vi "_readAppArgs.vi"(8 "error in (no error)":errorcluster, 11 "LVAutomationListener in":refnum<class "LVAutomationListener.lvclass">) -> (0 "error out":errorcluster, 3 "LVAutomationListener out":refnum<class "LVAutomationListener.lvclass">)   [LabVIEW 2013, in "LVAutomationListener.lvlib" / "LVAutomationListener.lvclass"]
doc: "Read the configuration file (if it exists) for values that will control this run of the application."
uses:
  LVAutomationListener.lvclass
  LVAutomationListener.lvclass/LVAutomationListener.ctl
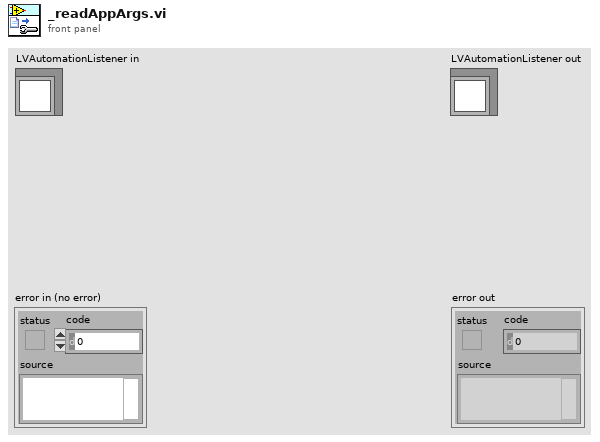
[diagram p1: front panel]
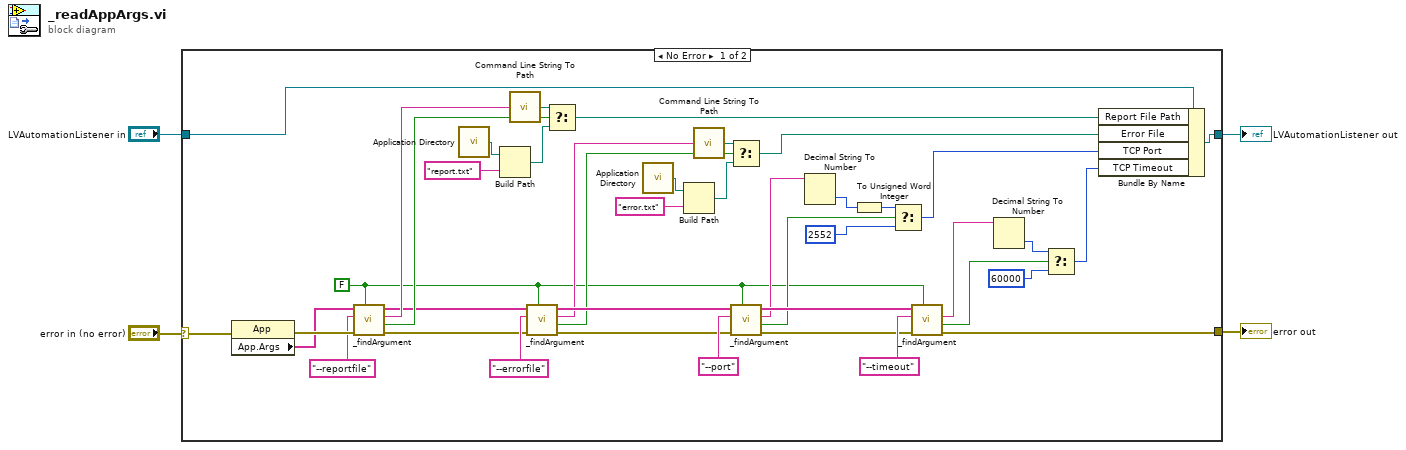
[diagram p0: block diagram]
diagram:
  n1 = case shown="No Error" "error in (no error)" {
    selector: "error in (no error)" -> [w46 w48]
    tunnel: [w21 w48] -> w3
    tunnel: [w43 w47] -> w1
    tunnel: "LVAutomationListener in" -> [w38 w47]
    frame No Error {
      w5 = FALSE ("Error If Not Found")
      n2 = property class="App"(error in=w46) -> (error out=w45:errorcluster, "App.Args"=w39:string[])  [unwired: 1 in, 1 out]
      n3 = call "_findArgument.vi"("Error If Not Found"=w5, "error in (no error)"=w45, "Argument"="--reportfile", "Arguments In"=w39) -> ("error out"=w15:errorcluster, "Found"=w40:bool, "Value"=w37:string, "Arguments Out"=w16:string[])  [unwired: 4 in]
      n4 = call <vilib>:"Application Directory.vi"() -> ("Application Directory"=w35:path)
      n5 = Build Path(base path=w35, name or relative path="report.txt") -> (appended path=w34:path)
      n6 = call <vilib>:"Command Line String To Path.vi"("string"=w37) -> ("path"=w36:path)
      n7 = call "_findArgument.vi"("Error If Not Found"=w5, "error in (no error)"=w15, "Argument"="--errorfile", "Arguments In"=w16) -> ("error out"=w13:errorcluster, "Found"=w7:bool, "Value"=w8:string, "Arguments Out"=w14:string[])  [unwired: 4 in]
      n8 = Select(t=w36, s=w40, f=w34) -> (s? t:f=w33:path)
      n9 = call <vilib>:"Application Directory.vi"() -> ("Application Directory"=w10:path)
      n10 = Build Path(base path=w10, name or relative path="error.txt") -> (appended path=w9:path)
      n11 = call <vilib>:"Command Line String To Path.vi"("string"=w8) -> ("path"=w11:path)
      n12 = Select(t=w11, s=w7, f=w9) -> (s? t:f=w6:path)
      n13 = call "_findArgument.vi"("Error If Not Found"=w5, "error in (no error)"=w13, "Argument"="--port", "Arguments In"=w14) -> ("error out"=w30:errorcluster, "Found"=w29:bool, "Value"=w28:string, "Arguments Out"=w31:string[])  [unwired: 4 in]
      n14 = Decimal String To Number(string=w28) -> (number=w18:i32)  [unwired: 2 in, 1 out]
      n15 = To Unsigned Word Integer(number=w18) -> (unsigned 16bit integer=w19:u16)
      n16 = Select(t=w19, s=w29, f=u16 2552) -> (s? t:f=w26:u16)
      n17 = call "_findArgument.vi"("Error If Not Found"=w5, "error in (no error)"=w30, "Argument"="--timeout", "Arguments In"=w31) -> ("error out"=w21:errorcluster, "Found"=w22:bool, "Value"=w23:string)  [unwired: 4 in, 1 out]
      n18 = Decimal String To Number(string=w23) -> (number=w25:i32)  [unwired: 2 in, 1 out]
      n19 = Select(t=w25, s=w22, f=60000) -> (s? t:f=w20:i32)
      n20 = Bundle By Name(cluster=w38, "Report File Path"=w33, "Error File"=w6, "TCP Port"=w26, "TCP Timeout"=w20) -> (w43:refnum<class "LVAutomationListener.lvclass">)
    }
    frame Error {
    }
  }
  "error out" <- w3
  "LVAutomationListener out" <- w1
